vi "GetColorDis.vi"() -> ()   [LabVIEW 2011]
uses:
  API/ColorSensorlib.lvlib
panel:
  out "返回值":bool
  in  "端口号":i32
  out "B值":i32
  out "G值":i32
  out "R值":i32
  in  "获取RGB按钮":bool
  in  "退出按钮":bool
  in  "初始化按钮":bool
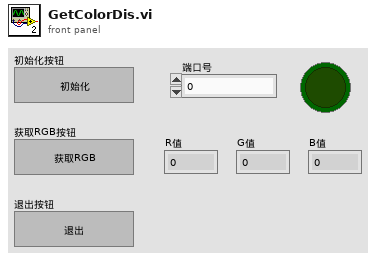
[diagram p1: front panel]
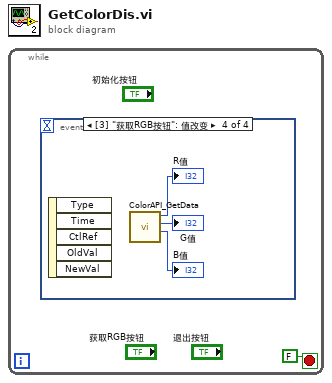
[diagram p0: block diagram]
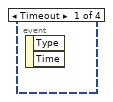
[diagram p2: hidden frame]
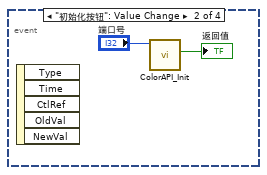
[diagram p3: hidden frame]
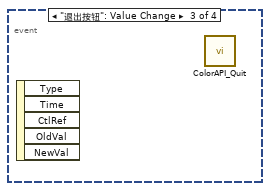
[diagram p4: hidden frame]
diagram:
  n1 = while {
    stop <- FALSE stop-if-true
    n2 = event shown="[3] \"获取RGB按钮\": 值改变" {
      selector: _ -> [_ _ _ _]
      dyn-events: _ -> [_ _ _ _]
      timeout: _ -> [_ _ _ _]
      event Timeout {
        n3 = event-data() -> ()  [unwired: 1 in, 2 out]
      }
      event "初始化按钮": Value Change {
        n4 = event-data() -> ()  [unwired: 1 in, 5 out]
        n5 = call "ColorAPI_Init.vi"("端口号"="端口号") -> ("返回值"=→"返回值":bool)  [unwired: 8 in, 2 out]
      }
      event "退出按钮": Value Change {
        n6 = event-data() -> ()  [unwired: 1 in, 5 out]
        n7 = call "ColorAPI_Quit.vi"() -> ()  [unwired: 11 in, 1 out]
      }
      event "获取RGB按钮": Value Change {
        n8 = event-data() -> ()  [unwired: 1 in, 5 out]
        n9 = call "ColorAPI_GetData.vi"() -> ("Blue"=→"B值":i32, "Green"=→"G值":i32, "Red"=→"R值":i32)  [unwired: 8 in, 1 out]
      }
    }
  }
